vi "Scan Variant from String__ogtk.vi"(7 "Format String (optional)":string, 8 "Default Value":variant, 9 "error in (no error)":errorcluster, 10 "Initial Scan Location":u32, 11 "Input String":string) -> (0 "Output":variant, 1 "error out":errorcluster, 2 "Offset Past Scan":u32, 3 "Remaining String":string)   [LabVIEW 2017]
doc: "Overcomes a limitation of \"Scan From String\" by allowing variant data types to be used/returned. This VI supports variant data for all LabVIEW data types supported by \"Scan From String\". \n\n<b>Notes:</b>\n<b>Format string</b> input may optionally be passed as a variant attribute named \"Format String\".\n<b>ISO 8601</b> is used as the default formating for Timestamp unless otherwise specified. <b>Timestamp</b> data must use the <b>Format String:</b> %T (or variations of %T), otherwise it will return an error."
panel:
  # "Scan Variant From String.vi\n\nPlease visit http://www.OpenG.org to learn about the\nOpen Source LabVIEW software movement.\n\nNOTICE -- YOU MUST LEAVE THIS NOTICE IN PLACE.  PER THE TERMS OF THE LICENSE BELOW, YOU MAY SUBLICENSE THIS SOFTWARE \nIN ANY WAY THAT DOES NOT CONFLICT WITH THIS LICENSE.\n\n### BSD License (http://www.opensource.org/licenses/bsd-license.php) Begin ###\n \nCopyright (c) 2002-2004, Jim Kring <jim@jimkring.com>\nCopyright (c) 2004, Michael C. Ashe <michael.ashe@imaginatics.com>\nCopyright (c) 2011, Jonathon Green <jg@jgcode.net>\nCopyright (c) 2011, Phillip Brooks <pbrooks100@gmail.com>\nCopyright (c) 2011, Jonas Mellroth<jonas.mellroth@wireflow.se>\n\nAll rights reserved.\n\nRedistribution and use in source and binary forms, with or without modification, are permitted provided that the following conditions are met:\n\n    * Redistributions of source code must retain the above copyright notice, this list of conditions and the following disclaimer.\n    * Redistributions in binary form must reproduce the above copyright notice, this list of conditions and the following disclaimer in the \n       documentation and/or other materials provided with the distribution.\n    * Neither the name of SciWare, James Kring, Inc., nor the names of its contributors may be used to endorse or promote products derived \n       from this software without specific prior written permission.\n\nTHIS SOFTWARE IS PROVIDED BY THE COPYRIGHT HOLDERS AND CONTRIBUTORS \"AS IS\" AND ANY EXPRESS OR IMPLIED WARRANTIES, \nINCLUDING, BUT NOT LIMITED TO, THE IMPLIED WARRANTIES OF MERCHANTABILITY AND FITNESS FOR A PARTICULAR PURPOSE ARE \nDISCLAIMED. IN NO EVENT SHALL THE COPYRIGHT OWNER OR CONTRIBUTORS BE LIABLE FOR ANY DIRECT, INDIRECT, INCIDENTAL,\n SPECIAL, EXEMPLARY, OR CONSEQUENTIAL DAMAGES (INCLUDING, BUT NOT LIMITED TO, PROCUREMENT OF SUBSTITUTE GOODS OR \nSERVICES; LOSS OF USE, DATA, OR PROFITS; OR BUSINESS INTERRUPTION) HOWEVER CAUSED AND ON ANY THEORY OF LIABILITY, \nWHETHER IN CONTRACT, STRICT LIABILITY, OR TORT (INCLUDING NEGLIGENCE OR OTHERWISE) ARISING IN ANY WAY OUT OF THE USE \nOF THIS SOFTWARE, EVEN IF ADVISED OF THE POSSIBILITY OF SUCH DAMAGE.\n\n### BSD License End ###"
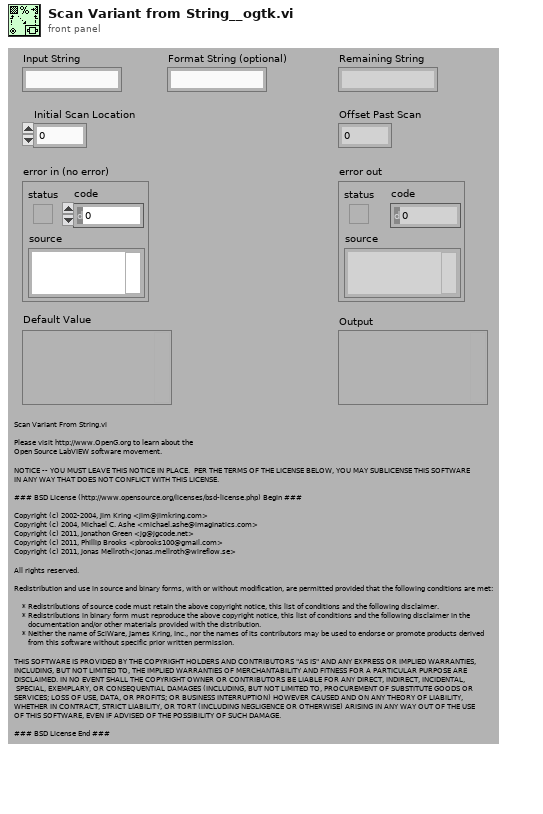
[diagram p1: front panel]
types:
  T1 = typedef "Type Descriptor Enumeration__ogtk.ctl" = enum8{"<Null>", "I8", "I16", "I32", "I64", "U8", "U16", "U32", "U64", "SGL", "DBL", "EXT", "CSG", "CDB", "CXT", "0x0F", "0x10", "0x11", "0x12", "0x13", "0x14", "Enum U8", "Enum U16", "Enum U32", "Enum U64", "SGL PQ", "DBL PQ", "EXT PQ", "CSG PQ", "CDB PQ", "CXT PQ", "0x1F", "0x20", "Boolean", "0x22", "0x23", "0x24", "0x25", "0x26", "0x27", "0x28", "0x29", "0x2A", "0x2B", "0x2C", "0x2D", "0x2E", "0x2F", "String", "0x31", "Path", "Pict", "0x34", "0x35", "0x36", "DAQ", "0x38", "0x39", "0x3A", "0x3B", "0x3C", "0x3D", "0x3E", "0x3F", "Array", "0x41", "0x42", "0x43", "0x44", "0x45", "0x46", "0x47", "0x48", "0x49", "0x4A", "0x4B", "0x4C", "0x4D", "0x4E", "0x4F", "Cluster", "0x51", "0x52", "Variant", "Waveform", "0x55", "0x56", "0x57", "0x58", "0x59", "0x5A", "0x5B", "0x5C", "0x5D", "0x5E", "0x5F", "0x60", "0x61", "0x62", "0x63", "0x64", "0x65", "0x66", "0x67", "0x68", "0x69", "0x6A", "0x6B", "0x6C", "0x6D", "0x6E", "0x6F", "Refnum"}
  T2 = typedef "Refnum Subtype Enum__ogtk.ctl" = enum8{"Generic", "Datalog File Refnum", "Byte Stream File Refnum", "Device Refnum", "Occurence Refnum", "TCP Connection Refnum", "VISA Refnum (Obsolete)", "Automation Renum", "VI Server Refnum", "Menu Refnum", "IVI Refnum (Obsolete)", "IMAQ Session", "0x0C", "Datasocket Refnum", "VISA Resource", "IVI Logical Name", "UDP Connection Refnum", "Notifier Refnum", "Queue Refnum", "IrDA Refnum", "Hardware Plugin Refnum", "Hardware Plugin Tag Refnum", "DAQmx Refnum", "Event Registration Refnum", ".NET Refnum", "User Event Refnum", "0x1A", "Event Callback", "0x1C", "0x1D", "Only Used Internal to LabVIEW", "Bluetooth", "Data Value References", "RT FIFO", "TDM Streaming"}
  T3 = typedef "Waveform Subtype Enum__ogtk.ctl" = enum8{"<Not a Waveform Type>", "0x01", "Analog 16-bit signed", "Analog Double-Precision", "0x04", "Analog Single Precision", "Timestamp", "Digital Data", "Digital Waveform", "Dynamic Data", "Analog Extended-Precision", "Analog 8-bit unsigned", "Analog 16-bit unsigned", "Analog 32-bit unsigned", "Analog 8-bit signed", "Analog 32-bit signed", "Analog Complex Single-Precision", "Analog Complex Double-Precision", "Analog Complex Extended Precision", "Analog 64-bit signed", "Analog 64-bit unsigned"}
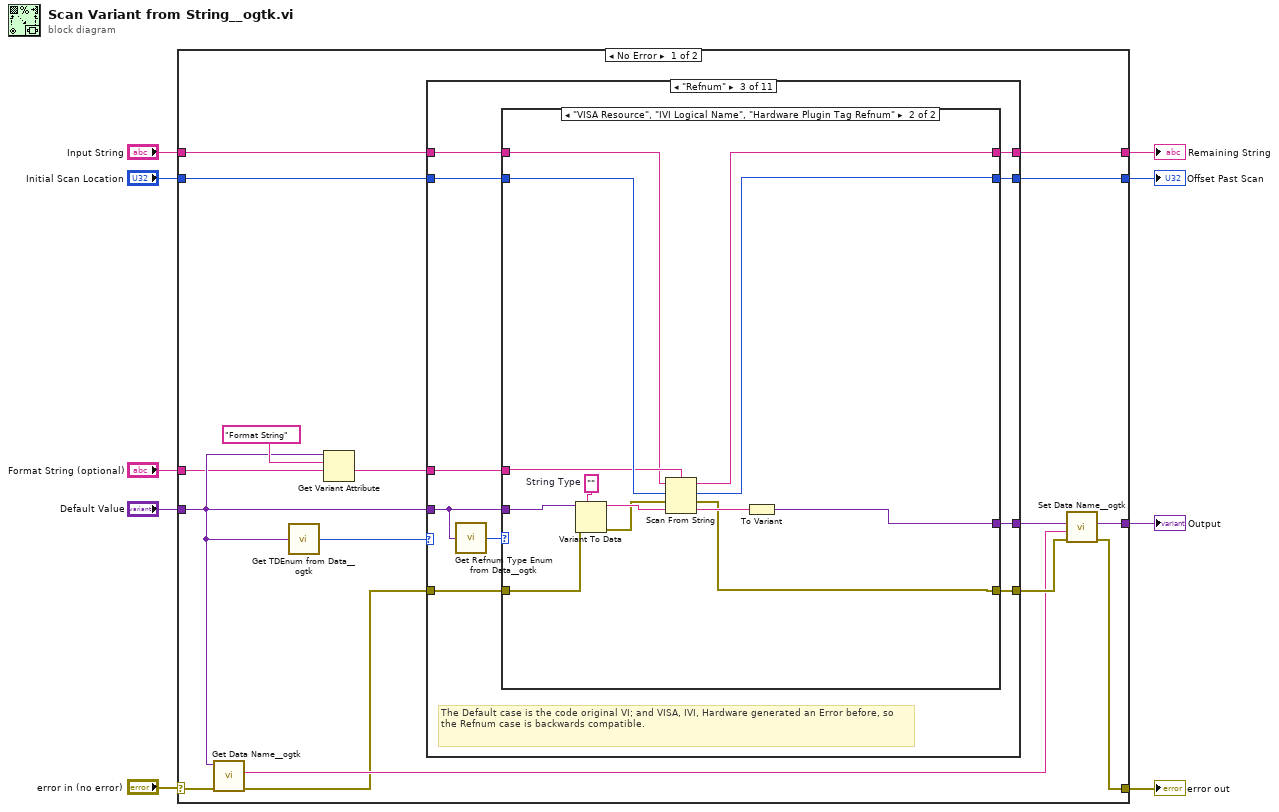
[diagram p0: block diagram]
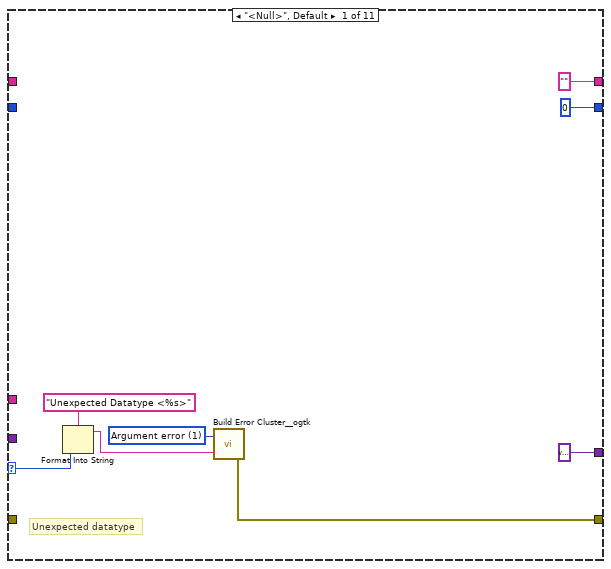
[diagram p2: hidden frame]
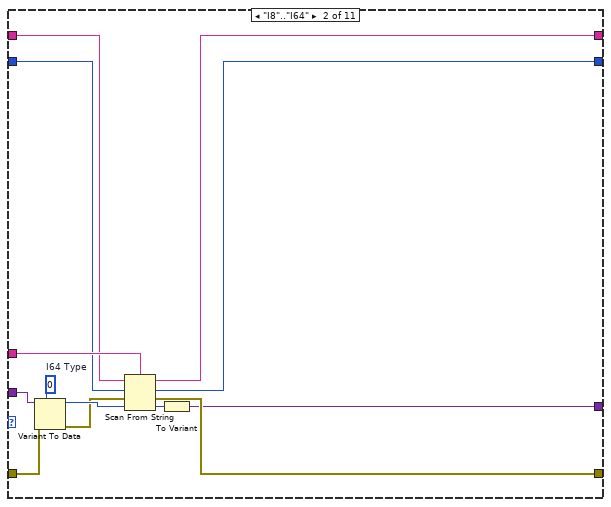
[diagram p3: hidden frame]
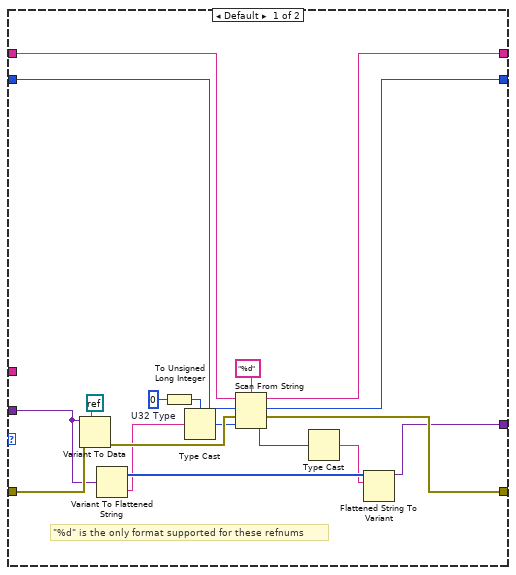
[diagram p4: hidden frame]
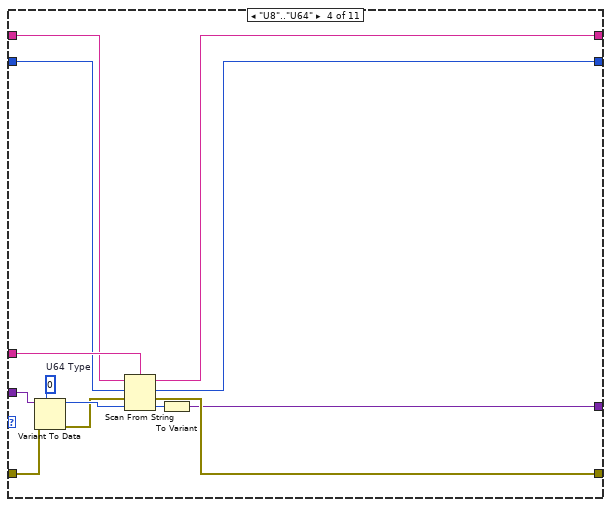
[diagram p5: hidden frame]
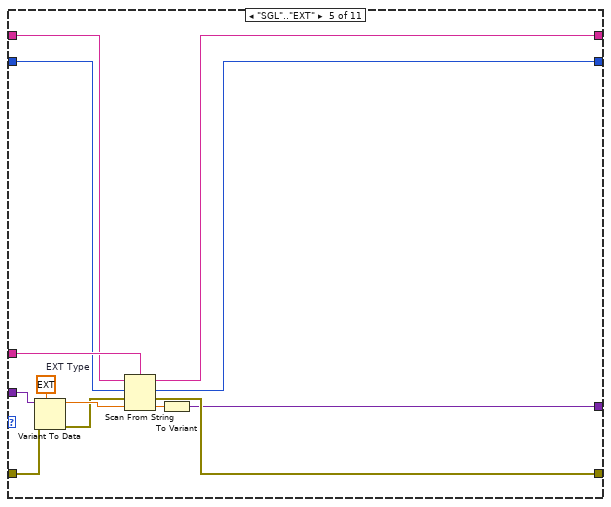
[diagram p6: hidden frame]
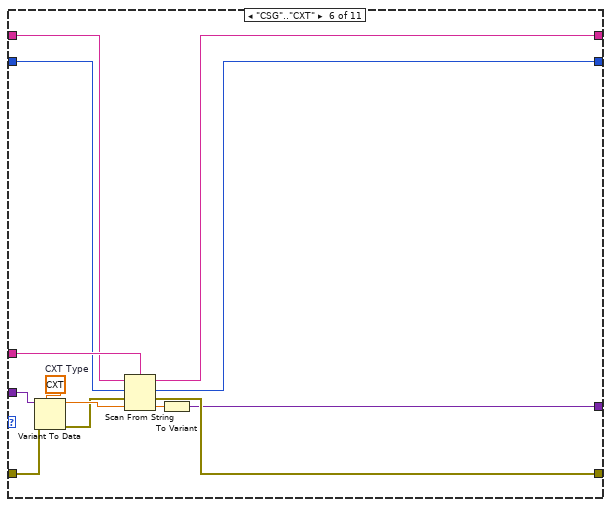
[diagram p7: hidden frame]
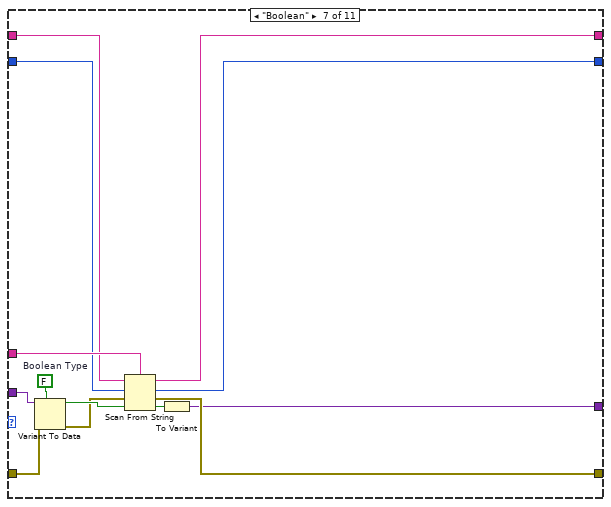
[diagram p8: hidden frame]
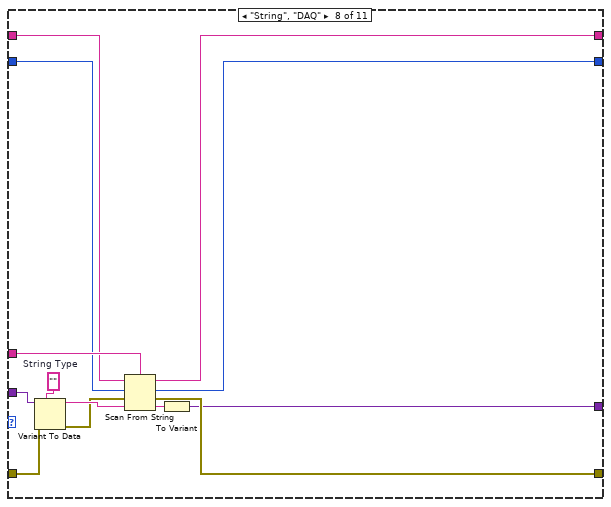
[diagram p9: hidden frame]
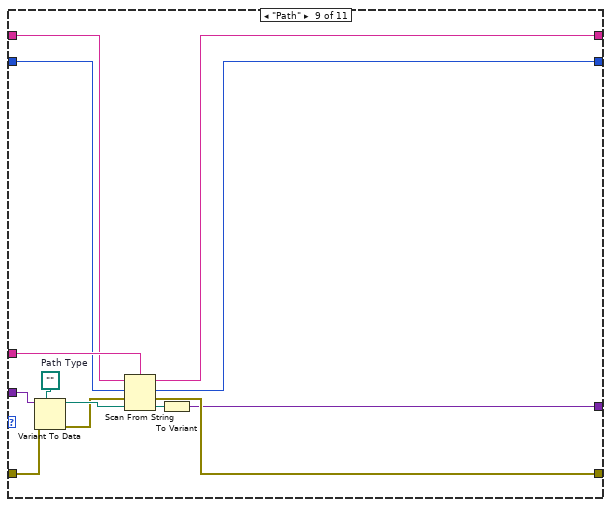
[diagram p10: hidden frame]
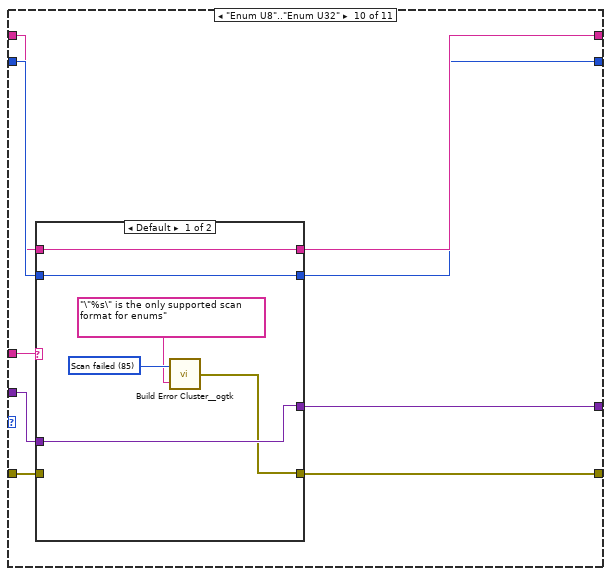
[diagram p11: hidden frame]
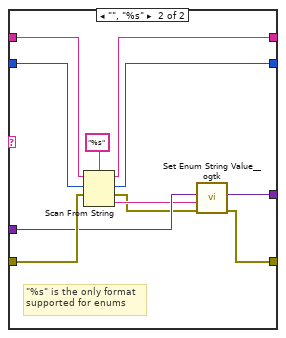
[diagram p12: hidden frame]
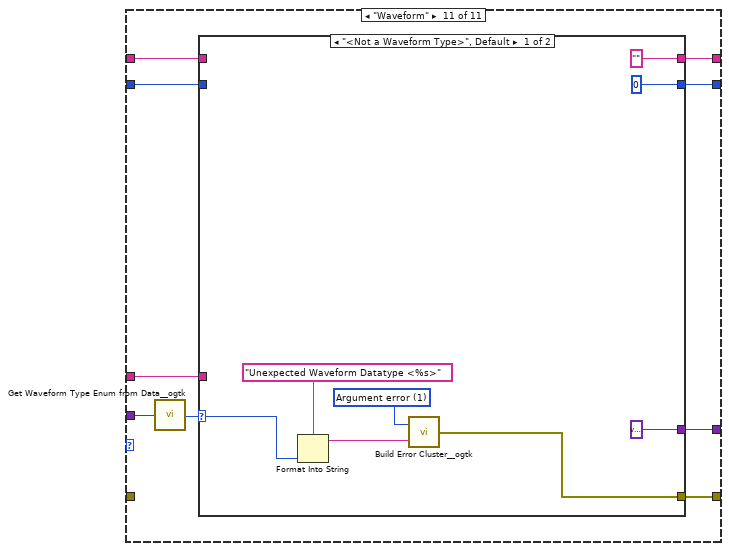
[diagram p13: hidden frame]
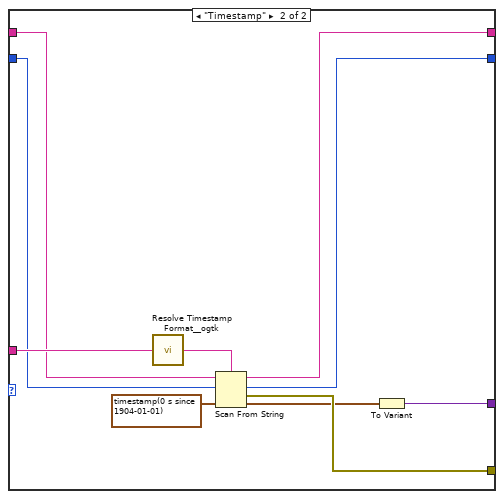
[diagram p14: hidden frame]
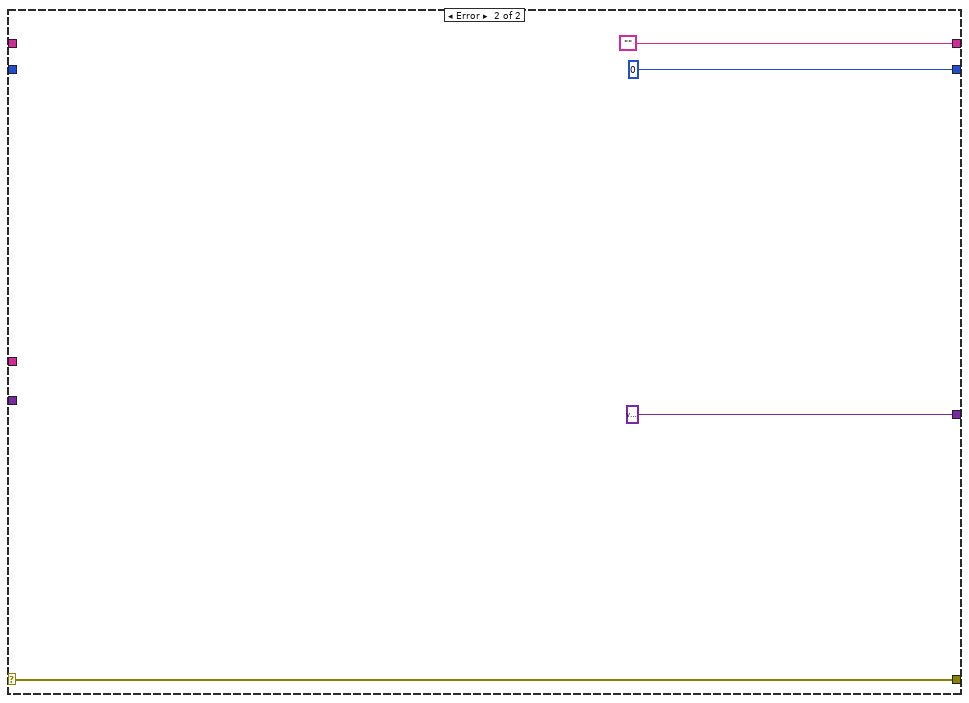
[diagram p15: hidden frame]
diagram:
  n1 = case shown="No Error" "error in (no error)" {
    selector: "error in (no error)" -> [w10 w222]
    tunnel: "Input String" -> [w24 _]
    tunnel: [w23 ""] -> w8
    tunnel: "Format String (optional)" -> [w14 _]
    tunnel: "Default Value" -> [w15 _]
    tunnel: [w18 w222] -> w4
    tunnel: "Initial Scan Location" -> [w22 _]
    tunnel: [w21 u32 0] -> w2
    tunnel: [w19 variant] -> w1
    frame No Error {
      n2 = call <userlib>:"Get Data Name__ogtk.vi"("error in (no error)"=w10, "Data"=w15) -> ("error out"=w11:errorcluster, "Data Name"=w16:string)  [unwired: 7 in, 1 out]
      n3 = call <userlib>:"Get TDEnum from Data__ogtk.vi"("Data"=w15) -> ("Type Descriptor Enumeration"=w12:T1)  [unwired: 4 in]
      n4 = Get Variant Attribute(Variant=w15, name="Format String", default value (empty Variant)=w14) -> (value=w13:string)  [unwired: 1 in, 3 out]
      n5 = case shown="\"Refnum\"" w12 {
        selector: w12 -> [w29 _ _ _ _ _ _ _ _ _ _]
        tunnel: w15 -> [_ w45 w48 w99 w112 w125 w138 w151 w164 w169 w200]
        tunnel: w13 -> [_ w44 w49 w98 w111 w124 w137 w150 w163 w166 w194]
        tunnel: [w28 w39 w53 w93 w106 w119 w132 w145 w158 w167 w198] -> w17
        tunnel: w11 -> [_ w43 w56 w97 w110 w123 w136 w149 w162 w174 _]
        tunnel: w24 -> [_ w41 w55 w95 w108 w121 w134 w147 w160 w172 w193]
        tunnel: ["" w40 w54 w94 w107 w120 w133 w146 w159 w171 w197] -> w23
        tunnel: w22 -> [_ w37 w52 w91 w104 w117 w130 w143 w156 w173 w192]
        tunnel: [u32 0 w36 w51 w90 w103 w116 w129 w142 w155 w170 w196] -> w21
        tunnel: [variant w34 w50 w88 w101 w114 w127 w140 w153 w168 w195] -> w20
        frame "<Null>", Default {
          w30 = 1 items=["No error", "Argument error", "Memory is full", "Out of zone", "End of file", "File already open", "Generic file I/O error", "File not found", "File permission error", "Disk is full", "Duplicate path", "Too many files open", "System feature not enabled", "Resource file not found", "Cannot add resource", "Resource not found", "Image not found", "Image memory error", "Pen does not exist", "Config type invalid", "Config token not found", "Config parse error", "Config memory error", "Bad external code format", "Bad external code offset", "External code not present", "Null window", "Destroy window error", "Null menu", "Print aborted", "Bad print record", "Print driver error", "Windows error during printing", "Memory error during printing", "Print dialog error", "Generic print error", "Invalid device refnum", "Device not found", "Device parameter error", "Device unit error", "Cannot open device", "Device call aborted", "Generic error", "Cancelled by user", "Object ID too low", "Object ID too high", "Object not in heap", "Unknown heap", "Unknown object (invalid DefProc)", "Unknown object (DefProc not in table)", "Message out of range", "Invalid (null) method", "Unknown message", "Manager call not supported", "Bad address", "Network operation in progress", "Network operation timed out", "Connection is busy", "Network attribute not supported", "Network error", "Address in use", "System out of memory", "Connection aborted", "Connection refused", "Not connected", "Already connected", "Connection closed", "Initialization error (interapplication manager)", "Bad occurrence", "Wait on unbound occurrence handler", "Occurrence queue overflow", "Datalog type conflict", "Unused", "Unrecognized type (interapplication manager)", "Memory corrupt", "Failed to make temporary DLL", "Old CIN version", "Drag socket not found", "Failed to load drop-object", "Failed to register OLE object", "Failed to release OLE object", "Format specifier type mismatch", "Unknown format specifier", "Too few format specifiers", "Too many format specifiers", "Scan failed", "Newer CIN version", "Error converting to variant", "Runtime menu error", "Password tampered", "Variant attribute not found", "Incompatible variant data type", "Event data is not available", "Event Store is not present", "Occurrence is not found", "Event Queue is not created", "Event info is not available", "Refnum passed is NULL", "Error retrieving Class GUID", "Error retrieving CoClass GUID", "Error retrieving TypeLib GUID.", "Bad built application magic bytes.", "Specific driver is different from the specific driver associated with the Logical Name.", "There is no session opened to the class driver.", "Max Error", "MAX - Error with config objects", "MAX - Error loading configuration", "MAX - Group not supported"]
          # "Unexpected datatype"
          n6 = Format Into String(format string="Unexpected Datatype <%s>" ("Format String"), w29) -> (resulting string=w32:string)  [unwired: 2 in, 1 out]
          n7 = call <userlib>:"Build Error Cluster__ogtk.vi"("String to Prepend to source (\"\")"=w32, "code"=w30) -> ("error out"=w28:errorcluster)
        }
        frame "I8".."I64" {
          w46 = i64 0  # I64 Type
          n8 = Variant To Data(error in=w43, type=w46, Variant=w45) -> (data=w42:i64, error out=w38:errorcluster)
          n9 = Scan From String(format string=w44, input string=w41, initial scan location=w37, error in=w38, default 1=w42) -> (remaining string=w40:string, offset past scan=w36:u32, error out=w39:errorcluster, output 1=w35:i64)
          n10 = To Variant(anything=w35) -> (Variant=w34:variant)
        }
        frame "Refnum" {
          # "The Default case is the code original VI; and VISA, IVI, Hardware generated an Error before, so the Refnum case is backwards compatible."
          n11 = call <userlib>:"Get Refnum Type Enum from Data__ogtk.vi"("Data"=w48) -> ("Refnum Subtype Enum"=w47:T2)  [unwired: 4 in]
          n12 = case shown="\"VISA Resource\", \"IVI Logical Name\", \"Hardware Plugin Tag Refnum\"" w47 {
            tunnel: w49 -> [_ w82]
            tunnel: w56 -> [w74 w84]
            tunnel: w55 -> [w73 w78]
            tunnel: [w72 w80] -> w54
            tunnel: [w71 w75] -> w53
            tunnel: w52 -> [w70 w83]
            tunnel: [w69 w81] -> w51
            tunnel: w48 -> [w68 w77]
            tunnel: [w67 w79] -> w50
            frame Default {
              w62 = u32 0  # U32 Type
              # "\"%d\" is the only format supported for these refnums"
              n13 = Variant To Data(error in=w74, type=refnum<k0> refnum, Variant=w68) -> (error out=w65:errorcluster)  [unwired: 1 out]
              n14 = Variant To Flattened String(Variant=w68) -> (data string=w59:string, 1:w60:i16[])
              n15 = To Unsigned Long Integer(number=w62) -> (unsigned 32bit integer=w61:u32)
              n16 = Type Cast(type=w61, x=w59) -> (*(type *) &x=w63:u32)
              n17 = Scan From String(format string="%d", input string=w73, initial scan location=w70, error in=w65, default 1=w63) -> (remaining string=w72:string, offset past scan=w69:u32, error out=w71:errorcluster, output 1=w64:u32)
              n18 = Type Cast(x=w64) -> (*(type *) &x=w58:string)  [unwired: 1 in]
              n19 = Flattened String To Variant(6:w58, 7:w60) -> (3:w67:variant)  [unwired: 1 in, 1 out]
            }
            frame "VISA Resource", "IVI Logical Name", "Hardware Plugin Tag Refnum" {
              w87 = ""  # String Type
              n20 = Variant To Data(error in=w84, type=w87, Variant=w77) -> (data=w86:string, error out=w85:errorcluster)
              n21 = Scan From String(format string=w82, input string=w78, initial scan location=w83, error in=w85, default 1=w86) -> (remaining string=w80:string, offset past scan=w81:u32, error out=w75:errorcluster, output 1=w76:string)
              n22 = To Variant(anything=w76) -> (Variant=w79:variant)
            }
          }
        }
        frame "U8".."U64" {
          w100 = u64 0  # U64 Type
          n23 = Variant To Data(error in=w97, type=w100, Variant=w99) -> (data=w96:u64, error out=w92:errorcluster)
          n24 = Scan From String(format string=w98, input string=w95, initial scan location=w91, error in=w92, default 1=w96) -> (remaining string=w94:string, offset past scan=w90:u32, error out=w93:errorcluster, output 1=w89:u64)
          n25 = To Variant(anything=w89) -> (Variant=w88:variant)
        }
        frame "SGL".."EXT" {
          w113 = ext 0.0  # EXT Type
          n26 = Variant To Data(error in=w110, type=w113, Variant=w112) -> (data=w109:ext, error out=w105:errorcluster)
          n27 = Scan From String(format string=w111, input string=w108, initial scan location=w104, error in=w105, default 1=w109) -> (remaining string=w107:string, offset past scan=w103:u32, error out=w106:errorcluster, output 1=w102:ext)
          n28 = To Variant(anything=w102) -> (Variant=w101:variant)
        }
        frame "CSG".."CXT" {
          w126 = cxt 0.0+0.0i  # CXT Type
          n29 = Variant To Data(error in=w123, type=w126, Variant=w125) -> (data=w122:cxt, error out=w118:errorcluster)
          n30 = Scan From String(format string=w124, input string=w121, initial scan location=w117, error in=w118, default 1=w122) -> (remaining string=w120:string, offset past scan=w116:u32, error out=w119:errorcluster, output 1=w115:cxt)
          n31 = To Variant(anything=w115) -> (Variant=w114:variant)
        }
        frame "Boolean" {
          w139 = FALSE  # Boolean Type
          n32 = Variant To Data(error in=w136, type=w139, Variant=w138) -> (data=w135:bool, error out=w131:errorcluster)
          n33 = Scan From String(format string=w137, input string=w134, initial scan location=w130, error in=w131, default 1=w135) -> (remaining string=w133:string, offset past scan=w129:u32, error out=w132:errorcluster, output 1=w128:bool)
          n34 = To Variant(anything=w128) -> (Variant=w127:variant)
        }
        frame "String", "DAQ" {
          w152 = ""  # String Type
          n35 = Variant To Data(error in=w149, type=w152, Variant=w151) -> (data=w148:string, error out=w144:errorcluster)
          n36 = Scan From String(format string=w150, input string=w147, initial scan location=w143, error in=w144, default 1=w148) -> (remaining string=w146:string, offset past scan=w142:u32, error out=w145:errorcluster, output 1=w141:string)
          n37 = To Variant(anything=w141) -> (Variant=w140:variant)
        }
        frame "Path" {
          w165 = path ""  # Path Type
          n38 = Variant To Data(error in=w162, type=w165, Variant=w164) -> (data=w161:path, error out=w157:errorcluster)
          n39 = Scan From String(format string=w163, input string=w160, initial scan location=w156, error in=w157, default 1=w161) -> (remaining string=w159:string, offset past scan=w155:u32, error out=w158:errorcluster, output 1=w154:path)
          n40 = To Variant(anything=w154) -> (Variant=w153:variant)
        }
        frame "Enum U8".."Enum U32" {
          n41 = case shown="Default" w166 {
            tunnel: w174 -> [_ w191]
            tunnel: w173 -> [w179 w190]
            tunnel: w172 -> [w180 w189]
            tunnel: [w180 w188] -> w171
            tunnel: [w179 w187] -> w170
            tunnel: w169 -> [w178 w186]
            tunnel: [w178 w184] -> w168
            tunnel: [w177 w182] -> w167
            frame Default {
              w176 = 85 items=["No error", "Argument error", "Memory is full", "Out of zone", "End of file", "File already open", "Generic file I/O error", "File not found", "File permission error", "Disk is full", "Duplicate path", "Too many files open", "System feature not enabled", "Resource file not found", "Cannot add resource", "Resource not found", "Image not found", "Image memory error", "Pen does not exist", "Config type invalid", "Config token not found", "Config parse error", "Config memory error", "Bad external code format", "Bad external code offset", "External code not present", "Null window", "Destroy window error", "Null menu", "Print aborted", "Bad print record", "Print driver error", "Windows error during printing", "Memory error during printing", "Print dialog error", "Generic print error", "Invalid device refnum", "Device not found", "Device parameter error", "Device unit error", "Cannot open device", "Device call aborted", "Generic error", "Cancelled by user", "Object ID too low", "Object ID too high", "Object not in heap", "Unknown heap", "Unknown object (invalid DefProc)", "Unknown object (DefProc not in table)", "Message out of range", "Invalid (null) method", "Unknown message", "Manager call not supported", "Bad address", "Network operation in progress", "Network operation timed out", "Connection is busy", "Network attribute not supported", "Network error", "Address in use", "System out of memory", "Connection aborted", "Connection refused", "Not connected", "Already connected", "Connection closed", "Initialization error (interapplication manager)", "Bad occurrence", "Wait on unbound occurrence handler", "Occurrence queue overflow", "Datalog type conflict", "Unused", "Unrecognized type (interapplication manager)", "Memory corrupt", "Failed to make temporary DLL", "Old CIN version", "Drag socket not found", "Failed to load drop-object", "Failed to register OLE object", "Failed to release OLE object", "Format specifier type mismatch", "Unknown format specifier", "Too few format specifiers", "Too many format specifiers", "Scan failed", "Newer CIN version", "Error converting to variant", "Runtime menu error", "Password tampered", "Variant attribute not found", "Incompatible variant data type", "Event data is not available", "Event Store is not present", "Occurrence is not found", "Event Queue is not created", "Event info is not available", "Refnum passed is NULL", "Error retrieving Class GUID", "Error retrieving CoClass GUID", "Error retrieving TypeLib GUID.", "Bad built application magic bytes.", "Specific driver is different from the specific driver associated with the Logical Name.", "There is no session opened to the class driver.", "Max Error", "MAX - Error with config objects", "MAX - Error loading configuration", "MAX - Group not supported"]
              n42 = call <userlib>:"Build Error Cluster__ogtk.vi"("String to Prepend to source (\"\")"="\"%s\" is the only supported scan format for enums" ("String to Prepend to source (\"\")"), "code"=w176) -> ("error out"=w177:errorcluster)
            }
            frame "", "%s" {
              # "\"%s\" is the only format\nsupported for enums"
              n43 = Scan From String(format string="%s" ("Format String"), input string=w189, initial scan location=w190, error in=w191) -> (remaining string=w188:string, offset past scan=w187:u32, error out=w183:errorcluster, output 1=w185:string)  [unwired: 1 in]
              n44 = call <userlib>:"Set Enum String Value__ogtk.vi"("error in (no error)"=w183, "String Value"=w185, "Default Enum Value"=w186) -> ("error out"=w182:errorcluster, "Enum"=w184:variant)  [unwired: 7 in]
            }
          }
        }
        frame "Waveform" {
          n45 = call <userlib>:"Get Waveform Type Enum from Data__ogtk.vi"("Data"=w200) -> ("Waveform Subtype Enum"=w199:T3)  [unwired: 4 in]
          n46 = case shown="\"<Not a Waveform Type>\", Default" w199 {
            selector: w199 -> [w201 _]
            tunnel: [w205 w216] -> w198
            tunnel: ["" w213] -> w197
            tunnel: [u32 0 w212] -> w196
            tunnel: [variant w215] -> w195
            tunnel: w194 -> [_ w217]
            tunnel: w193 -> [_ w210]
            tunnel: w192 -> [_ w209]
            frame "<Not a Waveform Type>", Default {
              w208 = 1 items=["No error", "Argument error", "Memory is full", "Out of zone", "End of file", "File already open", "Generic file I/O error", "File not found", "File permission error", "Disk is full", "Duplicate path", "Too many files open", "System feature not enabled", "Resource file not found", "Cannot add resource", "Resource not found", "Image not found", "Image memory error", "Pen does not exist", "Config type invalid", "Config token not found", "Config parse error", "Config memory error", "Bad external code format", "Bad external code offset", "External code not present", "Null window", "Destroy window error", "Null menu", "Print aborted", "Bad print record", "Print driver error", "Windows error during printing", "Memory error during printing", "Print dialog error", "Generic print error", "Invalid device refnum", "Device not found", "Device parameter error", "Device unit error", "Cannot open device", "Device call aborted", "Generic error", "Cancelled by user", "Object ID too low", "Object ID too high", "Object not in heap", "Unknown heap", "Unknown object (invalid DefProc)", "Unknown object (DefProc not in table)", "Message out of range", "Invalid (null) method", "Unknown message", "Manager call not supported", "Bad address", "Network operation in progress", "Network operation timed out", "Connection is busy", "Network attribute not supported", "Network error", "Address in use", "System out of memory", "Connection aborted", "Connection refused", "Not connected", "Already connected", "Connection closed", "Initialization error (interapplication manager)", "Bad occurrence", "Wait on unbound occurrence handler", "Occurrence queue overflow", "Datalog type conflict", "Unused", "Unrecognized type (interapplication manager)", "Memory corrupt", "Failed to make temporary DLL", "Old CIN version", "Drag socket not found", "Failed to load drop-object", "Failed to register OLE object", "Failed to release OLE object", "Format specifier type mismatch", "Unknown format specifier", "Too few format specifiers", "Too many format specifiers", "Scan failed", "Newer CIN version", "Error converting to variant", "Runtime menu error", "Password tampered", "Variant attribute not found", "Incompatible variant data type", "Event data is not available", "Event Store is not present", "Occurrence is not found", "Event Queue is not created", "Event info is not available", "Refnum passed is NULL", "Error retrieving Class GUID", "Error retrieving CoClass GUID", "Error retrieving TypeLib GUID.", "Bad built application magic bytes.", "Specific driver is different from the specific driver associated with the Logical Name.", "There is no session opened to the class driver.", "Max Error", "MAX - Error with config objects", "MAX - Error loading configuration", "MAX - Group not supported"]
              n47 = Format Into String(format string="Unexpected Waveform Datatype <%s>" ("Format String"), w201) -> (resulting string=w206:string)  [unwired: 2 in, 1 out]
              n48 = call <userlib>:"Build Error Cluster__ogtk.vi"("String to Prepend to source (\"\")"=w206, "code"=w208) -> ("error out"=w205:errorcluster)
            }
            frame "Timestamp" {
              n49 = call <userlib>:"Resolve Timestamp Format__ogtk.vi"("Timestamp Format In"=w217) -> ("Timestamp Format Out"=w211:string)
              n50 = Scan From String(format string=w211, input string=w210, initial scan location=w209, default 1=timestamp(0 s since 1904-01-01) ("Time Stamp")) -> (remaining string=w213:string, offset past scan=w212:u32, error out=w216:errorcluster, output 1=w214:timestamp)  [unwired: 1 in]
              n51 = To Variant(anything=w214) -> (Variant=w215:variant)
            }
          }
        }
      }
      n52 = call <userlib>:"Set Data Name__ogtk.vi"("error in (no error)"=w17, "Data Name"=w16, "Data"=w20) -> ("error out"=w18:errorcluster, "Renamed Data"=w19:variant)  [unwired: 7 in]
    }
    frame Error {
    }
  }
  "Remaining String" <- w8
  "error out" <- w4
  "Offset Past Scan" <- w2
  "Output" <- w1
